vi "Pre Launch Init.vi"(11 "GUARDAR_CSV in":refnum<class "GUARDAR_CSV.lvclass">) -> (0 "error out":errorcluster, 3 "GUARDAR_CSV out":refnum<class "GUARDAR_CSV.lvclass">)   [LabVIEW 2019, in "GUARDAR_CSV.lvlib" / "GUARDAR_CSV.lvclass"]
doc: "(<B>Filename</B>: Actor Framework.lvlib:Actor.lvclass:Pre Launch Init.vi)\n\nDefines behavior that occurs after the Launch Nested Actor method is invoked but before the actor's Actor Core method begins running.\n\nBy default, this method does nothing. A descendant class may override it to define behavior."
uses:
  GUARDAR_CSV.lvclass
  GUARDAR_CSV.lvclass/GUARDAR_CSV.ctl
  <vilib>/ActorFramework/Actor/Actor.lvclass
panel:
  in  "EXIT":bool=TRUE
  in  "GUARDAR?":bool=TRUE
  in  "DATO":string
  in  "PROVIENE DE?":enum16{"CONTADOR", "GENERADOR F"}(ring)
  in  "Path":path
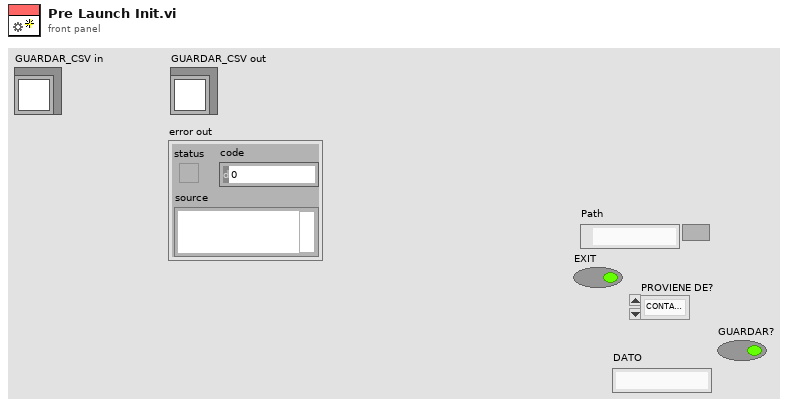
[diagram p1: front panel]
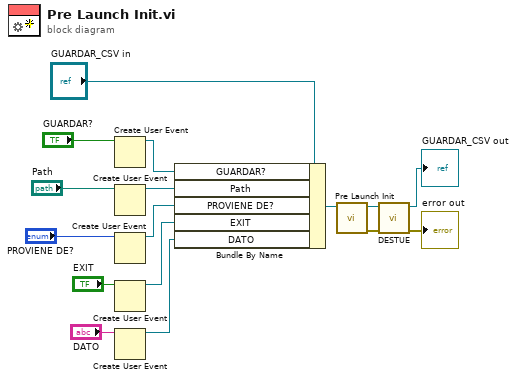
[diagram p0: block diagram]
diagram:
  n1 = Create User Event(user event datatype="GUARDAR?") -> (user event=w9:refnum<user-event>)  [unwired: 1 in, 1 out]
  n2 = Create User Event(user event datatype="Path") -> (user event=w8:refnum<user-event>)  [unwired: 1 in, 1 out]
  n3 = Create User Event(user event datatype="PROVIENE DE?") -> (user event=w7:refnum<user-event>)  [unwired: 1 in, 1 out]
  n4 = Create User Event(user event datatype="EXIT") -> (user event=w6:refnum<user-event>)  [unwired: 1 in, 1 out]
  n5 = Create User Event(user event datatype="DATO") -> (user event=w5:refnum<user-event>)  [unwired: 1 in, 1 out]
  n6 = Bundle By Name(cluster="GUARDAR_CSV in", "GUARDAR?"=w9, "Path"=w8, "PROVIENE DE?"=w7, "EXIT"=w6, "DATO"=w5) -> (w10:refnum<class "GUARDAR_CSV.lvclass">)
  n7 = call-parent "Pre Launch Init.vi"("Actor in"=w10) -> ("error out"=w4:errorcluster, "Actor out"=w3:refnum<class "GUARDAR_CSV.lvclass">)  [unwired: 9 in]
  n8 = call "DESTUE.vi"("error in (no error)"=w4, "GUARDAR_CSV in"=w3) -> ("error out"=→"error out":errorcluster, "GUARDAR_CSV out"=→"GUARDAR_CSV out":refnum<class "GUARDAR_CSV.lvclass">)  [unwired: 8 in]
